vi "FeedbackDecode_AllEMGHM.vi"(2 "Intensities":dbl[](array[numeric]), 3 "Mode":enum16{"Initialize", "Run"}(ring)) -> ()   [LabVIEW 2020]
panel:
  out "Stim":dbl[](array[numeric])
  out "Idxs":i32[](array[numeric])
  in  "HMSize":cluster{"NumCol":dbl, "NumRows":dbl}={"NumCol"=23.0, "NumRows"=22.0}
  out "EMGHM":picture
  out "EMGPos":T1={"[0]"=837, "[1]"=86, "[2]"=309, "[3]"=244}
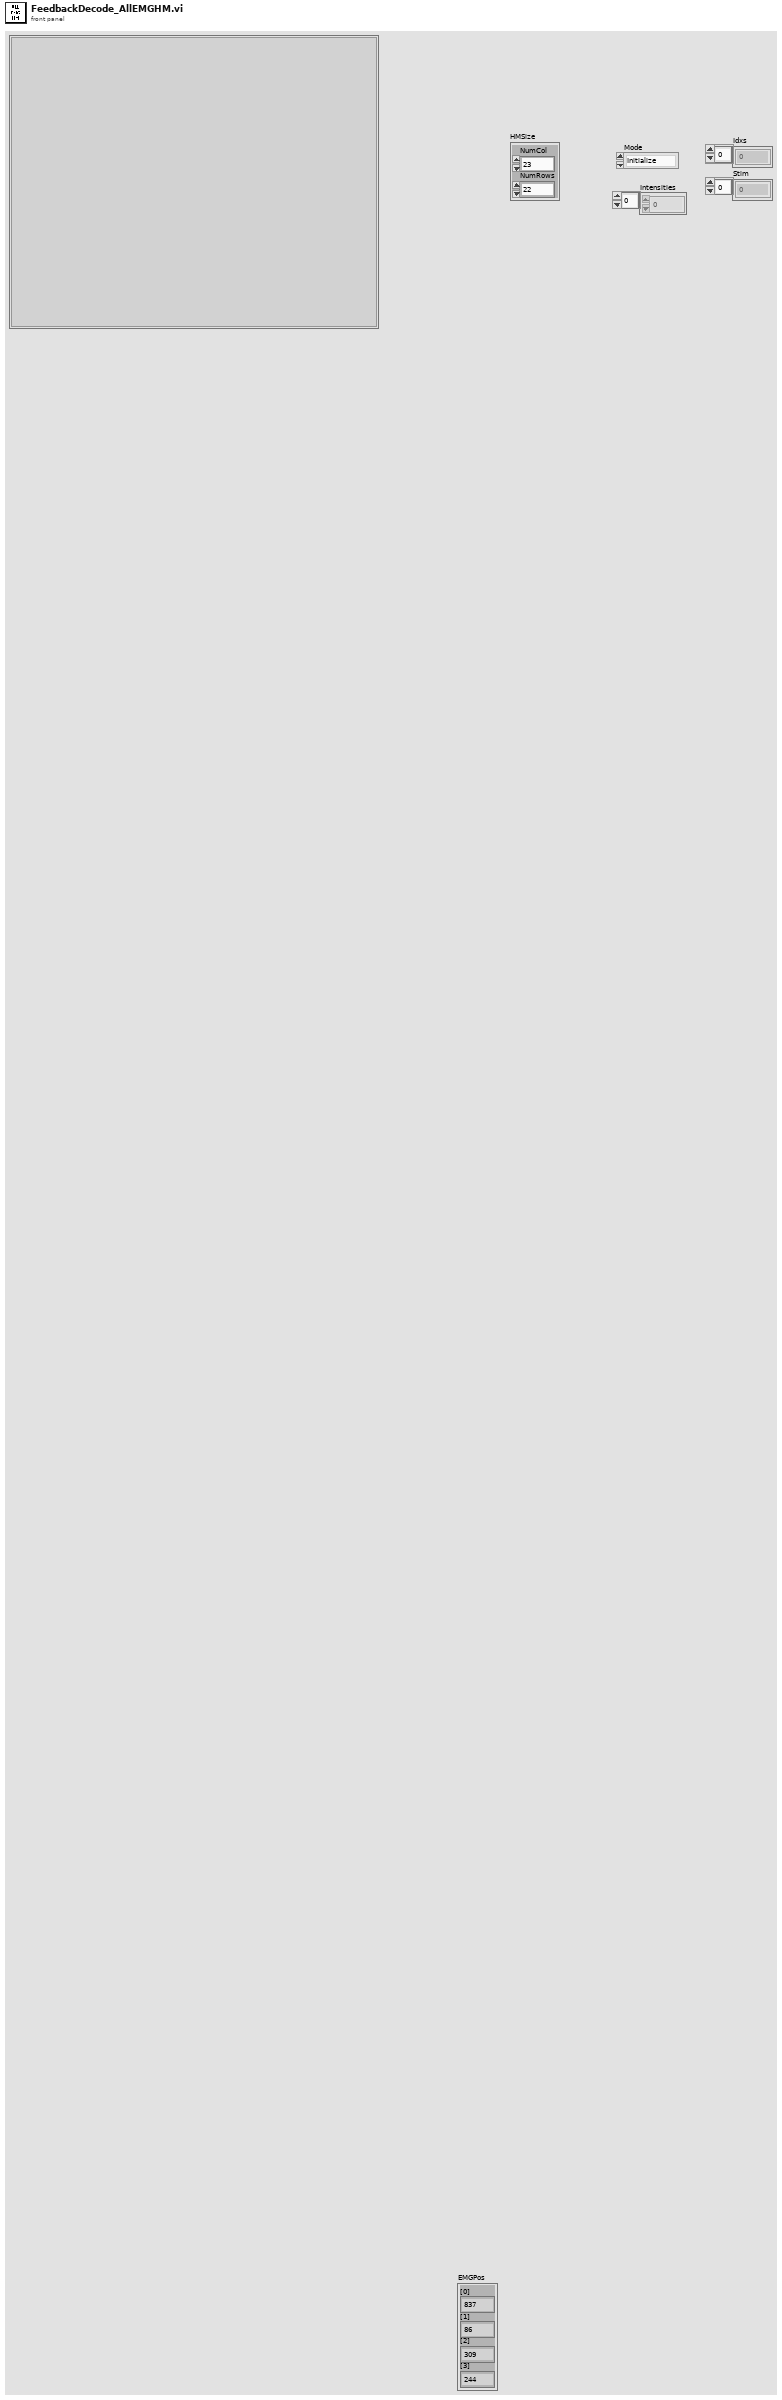
[diagram p1: front panel]
types:
  T1 = cluster{"[0]":u32, "[1]":u32, "[2]":u32, "[3]":u32}
  T2 = typedef "LVPositionTypeDef.ctl" = cluster{"Left":i32, "Top":i32}
  T3 = typedef "LVBoundsTypeDef.ctl" = cluster{"Width":u32, "Height":u32}
  T4 = cluster{cluster{"[0]":u32, "[1]":u32, "[2]":u32, "[3]":u32}, "HMSize":cluster{"NumCol":dbl, "NumRows":dbl}}
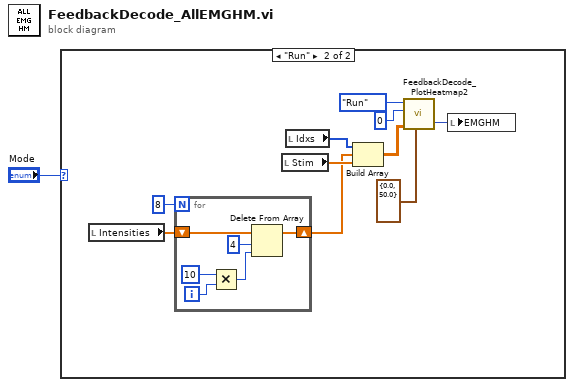
[diagram p0: block diagram]
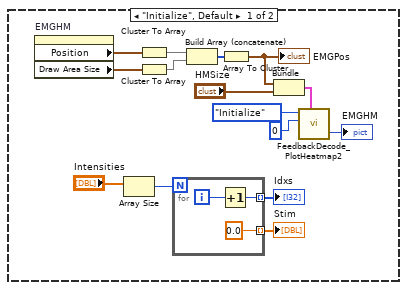
[diagram p2: hidden frame]
diagram:
  n1 = case shown="\"Run\"" "Mode" {
    frame "Initialize", Default {
      n2 = property on="EMGHM" class="Pict"() -> ("Position"=w8:T2, "Draw Area Size"=w7:T3)  [unwired: 2 in, 2 out]
      n3 = Array Size(array="Intensities") -> (size(s)=w3:i32)
      n4 = Cluster To Array(cluster=w8) -> (array=w11:i32[])
      n5 = Cluster To Array(cluster=w7) -> (array=w12:u32[])
      n6 = for {
        N: w3 -> [_]
        tunnel: [w18] -> w4 mode=indexing
        tunnel: [0.0] -> w5 mode=indexing
        i -> [w19]
        n7 = Increment(x=w19) -> (x+1=w18:i32)
      }
      "Idxs" <- w4
      "Stim" <- w5
      n8 = Build Array (concatenate)(w11, w12) -> (w13:u32[])
      n9 = Array To Cluster(array=w13) -> (cluster=w10:T1)
      "EMGPos" <- w10
      n10 = Bundle(w10, "HMSize"="HMSize") -> (w16:T4)  [unwired: 1 in]
      n11 = call "FeedbackDecode_PlotHeatmap2.vi"("InitCluster"=w16, "Instance"=0, "Mode"=enum16{"Initialize", "Run", "Mouse"}."Initialize") -> ("Pic"=→"EMGHM":picture)  [unwired: 3 in, 1 out]
    }
    frame "Run" {
      n12 = local read "Intensities"() -> (w22:dbl[])
      n13 = for {
        N: 8 -> [_]
        shift-right: [w30] -> w20
        shift-left: w22 -> [w31]
        i -> [w34]
        n14 = Multiply(x=10, y=w34) -> (x*y=w32:i32)
        n15 = Delete From Array(array=w31, length=4, index=w32) -> (array with subset deleted=w30:dbl[])  [unwired: 1 out]
      }
      n16 = local read "Stim"() -> (w25:dbl[])
      n17 = local read "Idxs"() -> (w26:i32[])
      n18 = Build Array(w26, w20, w25) -> (w24:dbl[][])
      n19 = call "FeedbackDecode_PlotHeatmap2.vi"("Range"=cluster{"Min":dbl, "Max":dbl} {"Min"=0.0, "Max"=50.0}, "GridIntensity"=w24, "Instance"=0, "Mode"=enum16{"Initialize", "Run", "Mouse"}."Run") -> ("Pic"=w29:picture)  [unwired: 2 in, 1 out]
      n20 = local write "EMGHM"(w29) -> ()
    }
  }
